vi "RSZVB Set A Wave Ideal Power Meter Match State.vi"(7 "State (Off)":bool, 8 "error in (no error)":errorcluster {"code" format="%.0x"}, 9 "Port Number (1)":i32=1, 10 "Channel (1)":i32=1, 11 "VISA session":refnum<visa-resource-name>) -> (0 "error out":errorcluster {"code" format="%.0x"}, 3 "dup VISA session":refnum<visa-resource-name>)   [LabVIEW 2011]
doc: "This VI enables or disables the assumption of an ideal power meter match when system error correction data and \npower calibration data are combined for the enhanced wave correction. \n\nRemote-control command(s):\n[SENSe<Ch>:]CORRection:POWer<port_no>:AWAVe:IPMMatch[:STATe]"
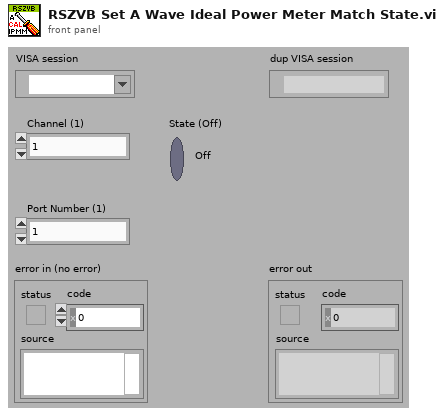
[diagram p1: front panel]
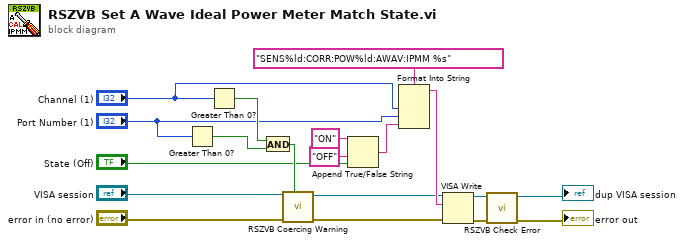
[diagram p0: block diagram]
diagram:
  n1 = Greater Than 0?(x="Port Number (1)") -> (x > 0?=w10:bool)
  n2 = Greater Than 0?(x="Channel (1)") -> (x > 0?=w12:bool)
  n3 = And(x=w12, y=w10) -> (x .and. y?=w11:bool)
  n4 = call "RSZVB Coercing Warning.vi"("In Range?"=w11, "error in (no error)"="error in (no error)", "VISA session"="VISA session") -> ("error out"=w8:errorcluster, "dup VISA session"=w9:refnum<visa-resource-name>)  [unwired: 7 in]
  n5 = Append True/False String(1:"State (Off)", 2:"OFF" ("false string"), 3:"ON" ("true string")) -> (0:w16:string)  [unwired: 1 in]
  n6 = Format Into String(format string="SENS%ld:CORR:POW%ld:AWAV:IPMM %s", "Channel (1)", "Port Number (1)", w16) -> (resulting string=w15:string)  [unwired: 2 in, 1 out]
  n7 = VISA Write(VISA resource name=w9, write buffer=w15, error in (no error)=w8) -> (VISA resource name out=w13:refnum<visa-resource-name>, error out=w14:errorcluster)  [unwired: 1 out]
  n8 = call "RSZVB Check Error.vi"("error in (no error)"=w14, "VISA session"=w13) -> ("error out"=→"error out":errorcluster, "dup VISA session"=→"dup VISA session":refnum<visa-resource-name>)  [unwired: 8 in]
